vi "Signal Destroy.vi"(8 "error in (no error)":errorcluster, 11 "Signal DVR in":refnum<data-value>) -> (0 "error out":errorcluster)   [LabVIEW 2012, in "MDSplus.lvlib"]
uses:
  <vilib>/MDSplus/Library/MDSplus.lvlib
  <vilib>/MDSplus/Classes/Data_Class/Compound_Class/Signal_Class/Signal.lvclass
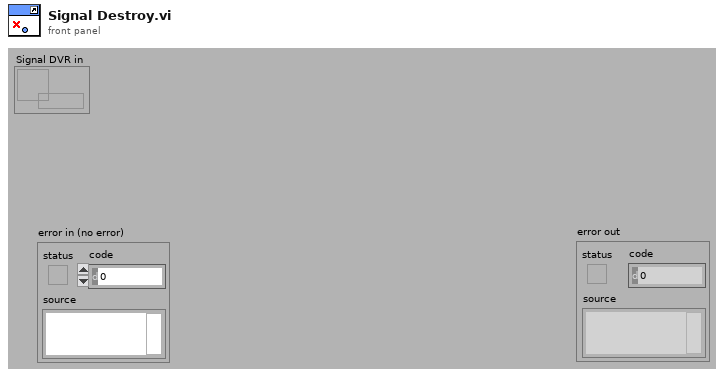
[diagram p1: front panel]
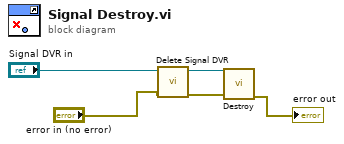
[diagram p0: block diagram]
diagram:
  n1 = call <vilib>:"Delete Signal DVR.vi"("error in (no error)"="error in (no error)", "Signal DVR in"="Signal DVR in") -> ("error out"=w2:errorcluster, "Signal out"=w1:refnum<class "Signal.lvclass">)  [unwired: 8 in]
  n2 = call-dynamic "Destroy.vi"("error in (no error)"=w2, "Signal in"=w1) -> ("error out"=→"error out":errorcluster)  [unwired: 9 in]
